vi "updateModel.vi"(8 "Error In":errorcluster, 11 "UI Elements Cluster":T1) -> (0 "Error Out":errorcluster)   [LabVIEW 2018]
uses:
  UI Module/src/controls/mainAppElementsCluster.ctl
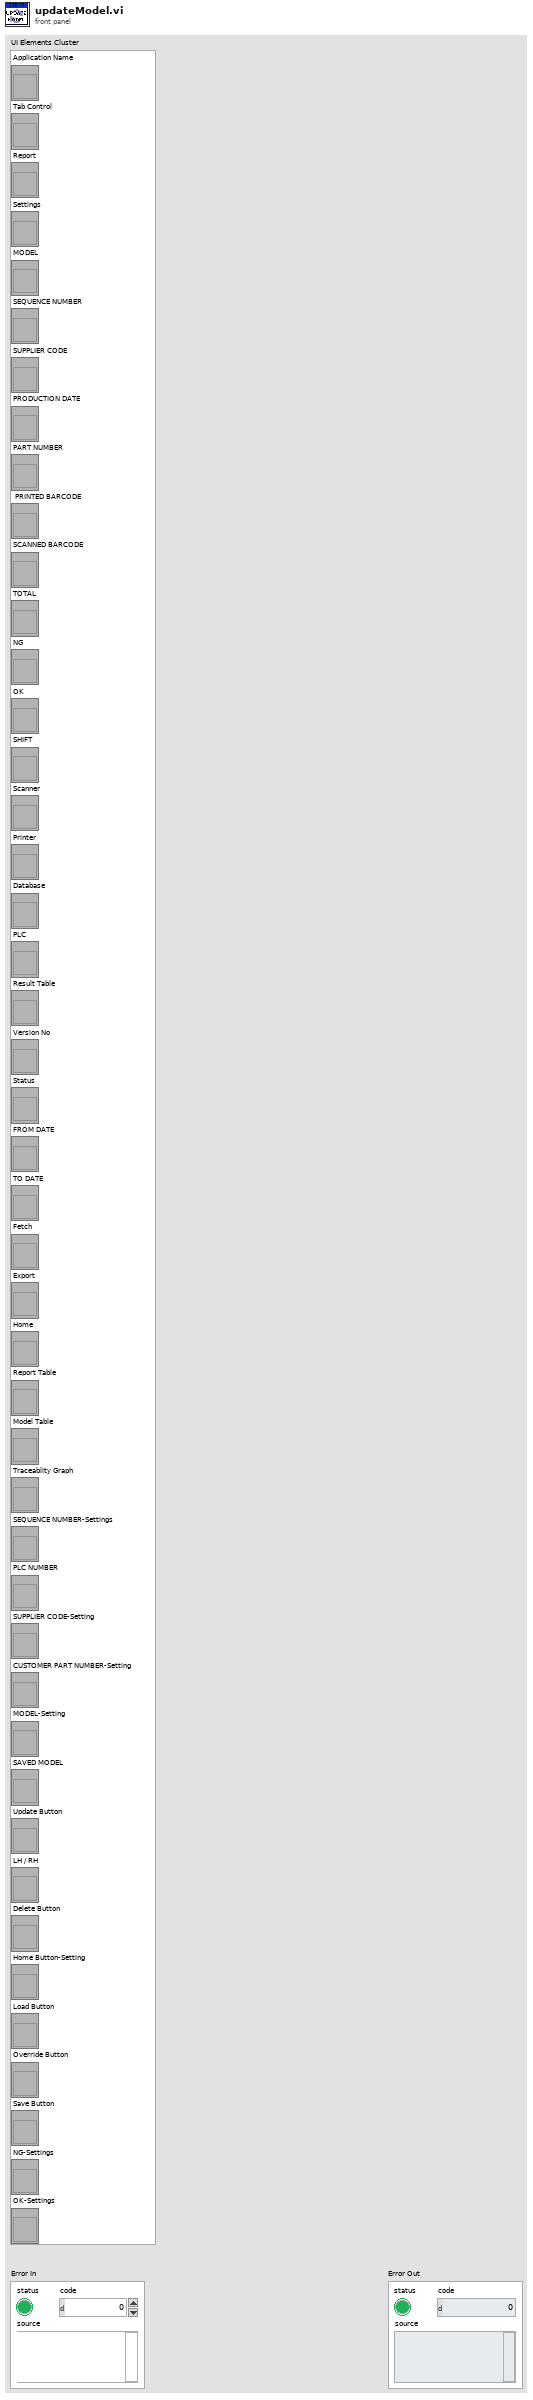
[diagram p1: front panel]
types:
  T1 = typedef "mainAppElementsCluster.ctl" = cluster{"Application Name":refnum<vi>, "Tab Control":refnum<vi>, "Status":refnum<vi>, "Version No":refnum<vi>, "Result Table":refnum<vi>, "PLC":refnum<vi>, "Database":refnum<vi>, "Printer":refnum<vi>, "Scanner":refnum<vi>, "SHIFT":refnum<vi>, "OK":refnum<vi>, "NG":refnum<vi>, "TOTAL":refnum<vi>, "SCANNED BARCODE":refnum<vi>, " PRINTED BARCODE":refnum<vi>, "PART NUMBER":refnum<vi>, "PRODUCTION DATE":refnum<vi>, "SUPPLIER CODE":refnum<vi>, "SEQUENCE NUMBER":refnum<vi>, "MODEL":refnum<vi>, "Settings":refnum<vi>, "Report":refnum<vi>, "Report Table":refnum<vi>, "Home":refnum<vi>, "Export":refnum<vi>, "Fetch":refnum<vi>, "TO DATE":refnum<vi>, "FROM DATE":refnum<vi>, "Model Table":refnum<vi>, "Traceablity Graph":refnum<vi>, "Override Button":refnum<vi>, "Load Button":refnum<vi>, "Home Button-Setting":refnum<vi>, "Delete Button":refnum<vi>, "Update Button":refnum<vi>, "Save Button":refnum<vi>, "SEQUENCE NUMBER-Settings":refnum<vi>, "PLC NUMBER":refnum<vi>, "LH / RH":refnum<vi>, "SUPPLIER CODE-Setting":refnum<vi>, "CUSTOMER PART NUMBER-Setting":refnum<vi>, "MODEL-Setting":refnum<vi>, "SAVED MODEL":refnum<vi>, "NG-Settings":refnum<vi>, "OK-Settings":refnum<vi>}
  T2 = cluster{"[0]":string, "[1]":string, "[2]":string, "[3]":string, "[4]":string, "[5]":string, "[6]":string, "[7]":string, "[8]":string}
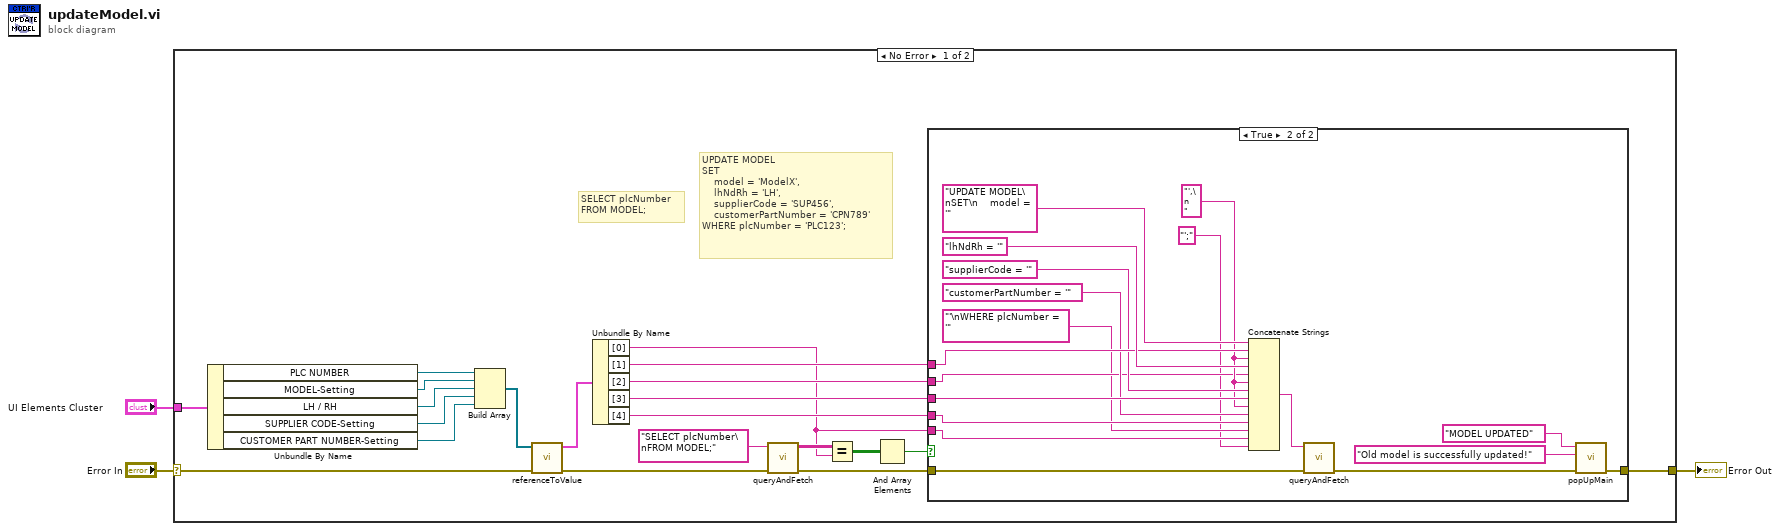
[diagram p0: block diagram]
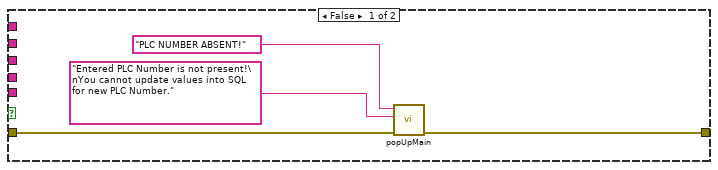
[diagram p2: hidden frame]
diagram:
  n1 = case shown="No Error" "Error In" {
    selector: "Error In" -> [w16 w47]
    tunnel: [w10 w47] -> w2
    tunnel: "UI Elements Cluster" -> [w24 _]
    frame No Error {
      # "SELECT plcNumber\nFROM MODEL;"
      # "UPDATE MODEL\nSET\n    model = 'ModelX',\n    lhNdRh = 'LH',\n    supplierCode = 'SUP456',\n    customerPartNumber = 'CPN789'\nWHERE plcNumber = 'PLC123';"
      n2 = Unbundle By Name(w24) -> ("PLC NUMBER"=w23:refnum<vi>, "MODEL-Setting"=w22:refnum<vi>, "LH / RH"=w21:refnum<vi>, "SUPPLIER CODE-Setting"=w20:refnum<vi>, "CUSTOMER PART NUMBER-Setting"=w19:refnum<vi>)
      n3 = Build Array(w23, w22, w21, w20, w19) -> (w18:refnum<vi>[])
      n4 = call "referenceToValue.vi"("Error In"=w16, "Reference Array"=w18) -> ("Error Out"=w15:errorcluster, "Value Out Cluster"=w17:T2)  [unwired: 8 in]
      n5 = Unbundle By Name(w17) -> ("[0]"=w4:string, "[1]"=w8:string, "[2]"=w7:string, "[3]"=w6:string, "[4]"=w5:string)
      n6 = call "queryAndFetch.vi"("Error In"=w15, "Query"="SELECT plcNumber\nFROM MODEL;") -> ("Error Out"=w11:errorcluster, "Result Table"=w13:string[][])  [unwired: 8 in]
      n7 = Equal?(x=w13, y=w4) -> (x = y?=w12:bool[][])
      n8 = And Array Elements(Boolean array=w12) -> (logical AND=w9:bool)
      n9 = case shown="True" w9 {
        tunnel: w11 -> [w28 w46]
        tunnel: [w27 w29] -> w10
        tunnel: w8 -> [_ w42]
        tunnel: w7 -> [_ w37]
        tunnel: w6 -> [_ w40]
        tunnel: w5 -> [_ w36]
        tunnel: w4 -> [_ w34]
        frame False {
          n10 = call "popUpMain.vi"("Error In"=w28, "Message Description"="Entered PLC Number is not present!\nYou cannot update values into SQL for new PLC Number." ("Error Info"), "Message Titlt"="PLC NUMBER ABSENT!" ("Error Name")) -> ("Error Out"=w27:errorcluster)  [unwired: 7 in, 1 out]
        }
        frame True {
          w39 = "',\n    "
          n11 = Concatenate Strings("UPDATE MODEL\nSET\n    model = '", w42, w39, "lhNdRh = '", w37, w39, "supplierCode = '", w40, w39, "customerPartNumber = '", w36, "'\nWHERE plcNumber = '", w34, "';") -> (w45:string)
          n12 = call "queryAndFetch.vi"("Error In"=w46, "Query"=w45) -> ("Error Out"=w30:errorcluster)  [unwired: 8 in, 1 out]
          n13 = call "popUpMain.vi"("Error In"=w30, "Message Description"="Old model is successfully updated!" ("Error Info"), "Message Titlt"="MODEL UPDATED" ("Error Name")) -> ("Error Out"=w29:errorcluster)  [unwired: 7 in, 1 out]
        }
      }
    }
    frame Error {
    }
  }
  "Error Out" <- w2
